vi "Read Show BD.vi"(8 "error in (no error)":errorcluster, 11 "AFM_Litho_Plugin.IV in":refnum<class "AFM_Litho_Plugin.IV.lvclass">) -> (0 "error out":errorcluster, 2 "Show BD":bool, 3 "AFM_Litho_Plugin.IV out":refnum<class "AFM_Litho_Plugin.IV.lvclass">)   [LabVIEW 2019, in "AFM_Litho_Plugin.IV.lvclass"]
uses:
  AFM_Litho_Plugin.IV.lvclass
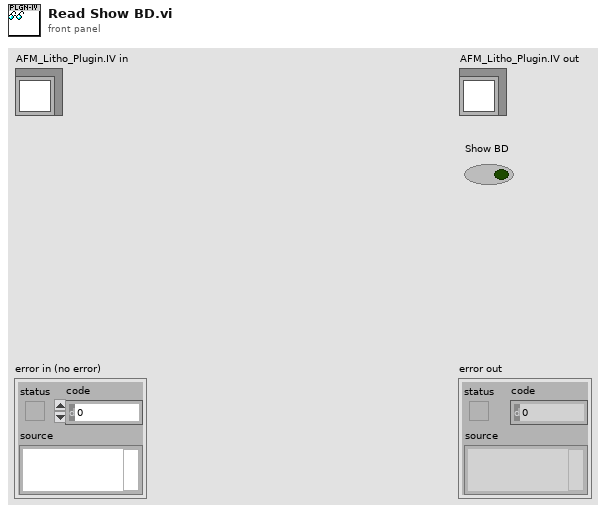
[diagram p1: front panel]
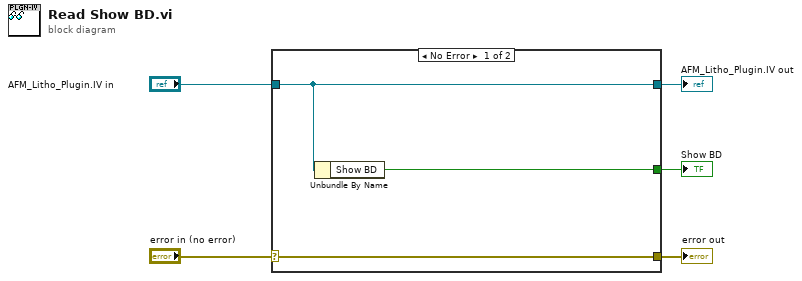
[diagram p0: block diagram]
diagram:
  n1 = case shown="No Error" "error in (no error)" {
    selector: "error in (no error)" -> [w8 w9]
    tunnel: [w8 w9] -> w4
    tunnel: [w7 w10] -> w2
    tunnel: "AFM_Litho_Plugin.IV in" -> [w7 w10]
    tunnel: [w6 _] -> w1
    frame No Error {
      n2 = Unbundle By Name(w7) -> ("Show BD"=w6:bool)
    }
    frame Error {
    }
  }
  "error out" <- w4
  "AFM_Litho_Plugin.IV out" <- w2
  "Show BD" <- w1
